vi "Read Associated Cells.vi"(8 "error in (no error)":errorcluster, 11 "Associated Data in":refnum<class "Associated Data.lvclass">) -> (0 "error out":errorcluster, 2 "Associated Cells":cluster{"PAS":dbl, "CRD":dbl}[](array[cluster]), 3 "Associated Data out":refnum<class "Associated Data.lvclass">)   [LabVIEW 2015, in "Associated Data.lvclass"]
uses:
  Associated Data.lvclass
  Associated Data.lvclass/Associated Data.ctl
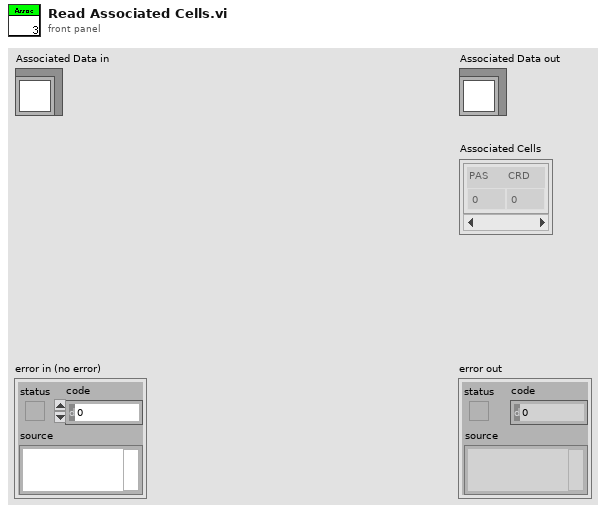
[diagram p1: front panel]
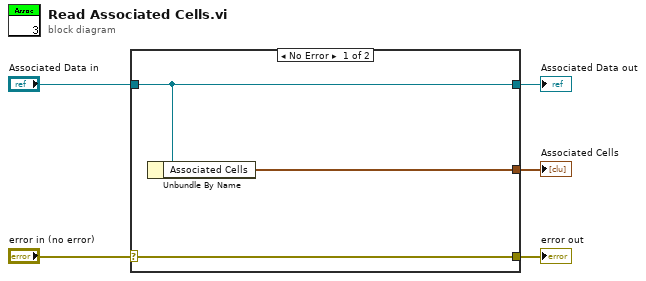
[diagram p0: block diagram]
diagram:
  n1 = case shown="No Error" "error in (no error)" {
    selector: "error in (no error)" -> [w8 w9]
    tunnel: [w8 w9] -> w4
    tunnel: [w7 w10] -> w2
    tunnel: "Associated Data in" -> [w7 w10]
    tunnel: [w6 _] -> w1
    frame No Error {
      n2 = Unbundle By Name(w7) -> ("Associated Cells"=w6:cluster{"PAS":dbl, "CRD":dbl}[])
    }
    frame Error {
    }
  }
  "error out" <- w4
  "Associated Data out" <- w2
  "Associated Cells" <- w1
